vi "TCP Server Listener Process Core.vi"(0 "TCP Server RefNum":refnum<class "JKI TCP Server.lvclass">) -> ()   [LabVIEW 2020, in "JKI TCP Server.lvclass"]
uses:
  JKI TCP Server.lvclass
  _Data Structures/TCP Server Connection Process Data Cluster.ctl
  TCP Server Connection Process.vi
  JKI TCP Server.lvclass/JKI TCP Server.ctl
panel:
  # "This VI Must Be Reentrant if multiple *servers* are to be created."
  # "Copyright © 2004-2008 JKI. All rights reserved.\n\nAuthor: Jim Kring [jim.kring@jameskring.com]\n\nThis library is provided \"AS IS\" ,WITHOUT WARRANTIES OR \nCONDITIONS OF ANY KIND, either express or implied.\n\nJames Kring, Inc. -- http://www.jameskring.com"
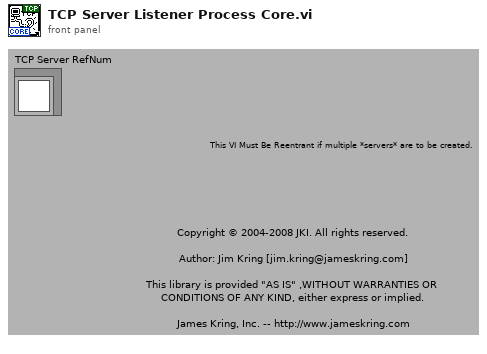
[diagram p1: front panel]
types:
  T1 = typedef "JKI TCP Server.lvclass/TCP Server Connection Process Data Cluster.ctl" = cluster{"connection ID":refnum<k5>, "remote address":string, "remote port":u16, "Connection Process VI Refnum":refnum<vi>, "Connection Start Time":u32}
  T2 = typedef "JKI TCP Server.lvclass/TCP Server Data.ctl" = cluster{"Listener Info":T3, "Connection Process VI RefNums":refnum<vi>[], "dup connection IDs (for quick search)":refnum<k5>[], "Connections":T4[], "Connection Handler VI Path":path, "Handler Is Reentrant?":bool, "TCP Handler Instance RefNums":T5[], "TCP Handler VI RefNum":T5, "No. Connections":u32, "Max Connections":u32, "server start time":u32, "Additional Data":variant}
  T3 = typedef "JKI TCP Server.lvclass/TCP Server Listener Info Cluster.ctl" = cluster{"listener ID":refnum<k5>, "net address":u32, "port":u16, "Listener Process VI Refnum":refnum<vi>}
  T4 = typedef "JKI TCP Server.lvclass/TCP Server Connection Info Cluster.ctl" = cluster{"connection ID":refnum<k5>, "Remote Address":string, "remote port":u16, "connection start time":u32}
  T5 = typedef "JKI TCP Server.lvclass/TCP Server Handler RefNum.ctl" = refnum<vi>
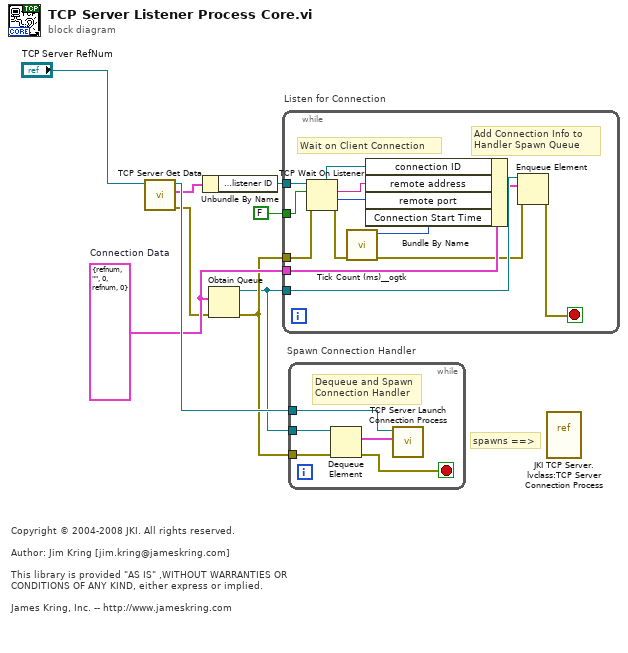
[diagram p0: block diagram]
diagram:
  w8 = T1 {"connection ID"=refnum, "remote address"="", "remote port"=0, "Connection Process VI Refnum"=refnum, "Connection Start Time"=0}  # Connection Data
  # "Copyright © 2004-2008 JKI. All rights reserved.\n\nAuthor: Jim Kring [jim.kring@jameskring.com]\n\nThis library is provided \"AS IS\" ,WITHOUT WARRANTIES OR \nCONDITIONS OF ANY KIND, either express or implied.\n\nJames Kring, Inc. -- http://www.jameskring.com"
  # "spawns ==>"
  n1 = call "TCP Server Get Data.vi"("TCP Server"="TCP Server RefNum") -> ("error out"=w6:errorcluster, "Data out"=w4:T2, "TCP Server out"=w9:refnum<class "JKI TCP Server.lvclass">)  [unwired: 8 in]
  n2 = Unbundle By Name(w4) -> ("Listener Info.listener ID"=w3:refnum<k5>)
  n3 = Obtain Queue(element data type=w8, error in (no error)=w6) -> (queue out=w5:refnum<queue>, error out=w7:errorcluster)  [unwired: 3 in, 1 out]
  n4 = while "Listen for Connection" {
    tunnel: w7 -> [w22]
    tunnel: w3 -> [w21]
    tunnel: w5 -> [w17]
    tunnel: w8 -> [w20]
    tunnel: FALSE ("resolve remote address (T)") -> [w10]
    stop <- w14 stop-if-true
    # "Add Connection Info to Handler Spawn Queue"
    # "Wait on Client Connection"
    n5 = TCP Wait On Listener(8:w22, 10:w10, 11:w21) -> (0:w13:errorcluster, 1:w19:u16, 2:w18:string, 4:w15:refnum<k5>)  [unwired: 1 in, 1 out]
    n6 = call <userlib>:"Tick Count (ms)__ogtk.vi"("error in (no error)"=w13) -> ("error out"=w12:errorcluster, "millisecond timer value"=w11:u32)  [unwired: 9 in]
    n7 = Bundle By Name(cluster=w20, "connection ID"=w15, "remote address"=w18, "remote port"=w19, "Connection Start Time"=w11) -> (w16:T1)
    n8 = Enqueue Element(queue=w17, element=w16, error in (no error)=w12) -> (error out=w14:errorcluster)  [unwired: 1 in, 2 out]
  }
  n9 = while "Spawn Connection Handler" {
    tunnel: w5 -> [w27]
    tunnel: w7 -> [w26]
    tunnel: w9 -> [w24]
    stop <- w23 stop-if-true
    # "Dequeue and Spawn Connection Handler"
    n10 = Dequeue Element(queue=w27, error in (no error)=w26) -> (element=w25:T1, error out=w23:errorcluster)  [unwired: 1 in, 2 out]
    n11 = call "TCP Server Launch Connection Process.vi"("Connection Data"=w25, "TCP Server RefNum"=w24) -> ()  [unwired: 9 in, 1 out]
  }
  n12 = vi-ref "JKI TCP Server.lvclass:TCP Server Connection Process.vi"() -> ()  [unwired: 1 out]
